vi "rad_GetImageVersionStatus.vi"(0 "Image Version":string, 5 "RAD Version":string, 11 "error in (no error)":errorcluster) -> (4 "Supported":bool, 6 "Current":bool, 8 "Older":bool, 10 "Newer":bool, 15 "error out":errorcluster)   [LabVIEW 2014]
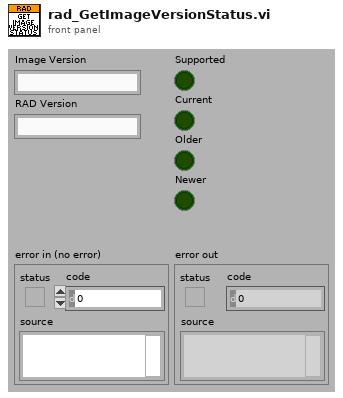
[diagram p1: front panel]
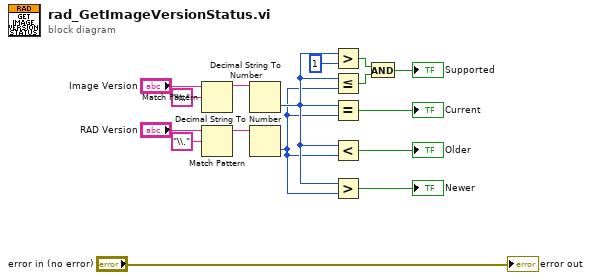
[diagram p0: block diagram]
diagram:
  n1 = Match Pattern(string="Image Version", regular expression="\\.") -> (before substring=w12:string)  [unwired: 1 in, 3 out]
  n2 = Match Pattern(string="RAD Version", regular expression="\\.") -> (before substring=w11:string)  [unwired: 1 in, 3 out]
  n3 = Decimal String To Number(string=w12) -> (number=w5:i32)  [unwired: 2 in, 1 out]
  n4 = Decimal String To Number(string=w11) -> (number=w4:i32)  [unwired: 2 in, 1 out]
  n5 = Greater?(x=w5, y=1) -> (0:w2:bool)
  n6 = Less Or Equal?(x=w5, y=w4) -> (x <= y?=w1:bool)
  n7 = Equal?(x=w5, y=w4) -> (x = y?=→"Current":bool)
  n8 = Less?(x=w5, y=w4) -> (x < y?=→"Older":bool)
  n9 = Greater?(x=w5, y=w4) -> (0:→"Newer":bool)
  n10 = And(x=w2, y=w1) -> (x .and. y?=→"Supported":bool)
  "error out" <- "error in (no error)"
